vi "storeADCMixedToArray-vphil.vi"(2 "dataBlockArray1":string[](array[string]), 3 "ADCselect":enum16{"ADC18", "ADC16", "2ADC", "None"}(ring)) -> (0 "ADC16Resets":i32, 1 "TotalTrigger":i32)   [LabVIEW 2014]
uses:
  Global 1.vi
panel:
  out "ADC18Resets":i32
  out "ADC18Counter":i32
  out "ADC16Counter":i32
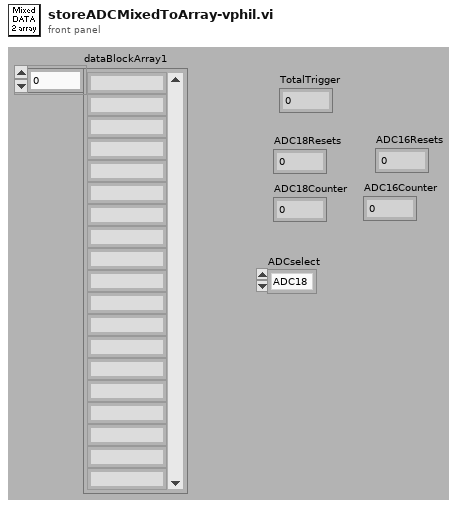
[diagram p1: front panel]
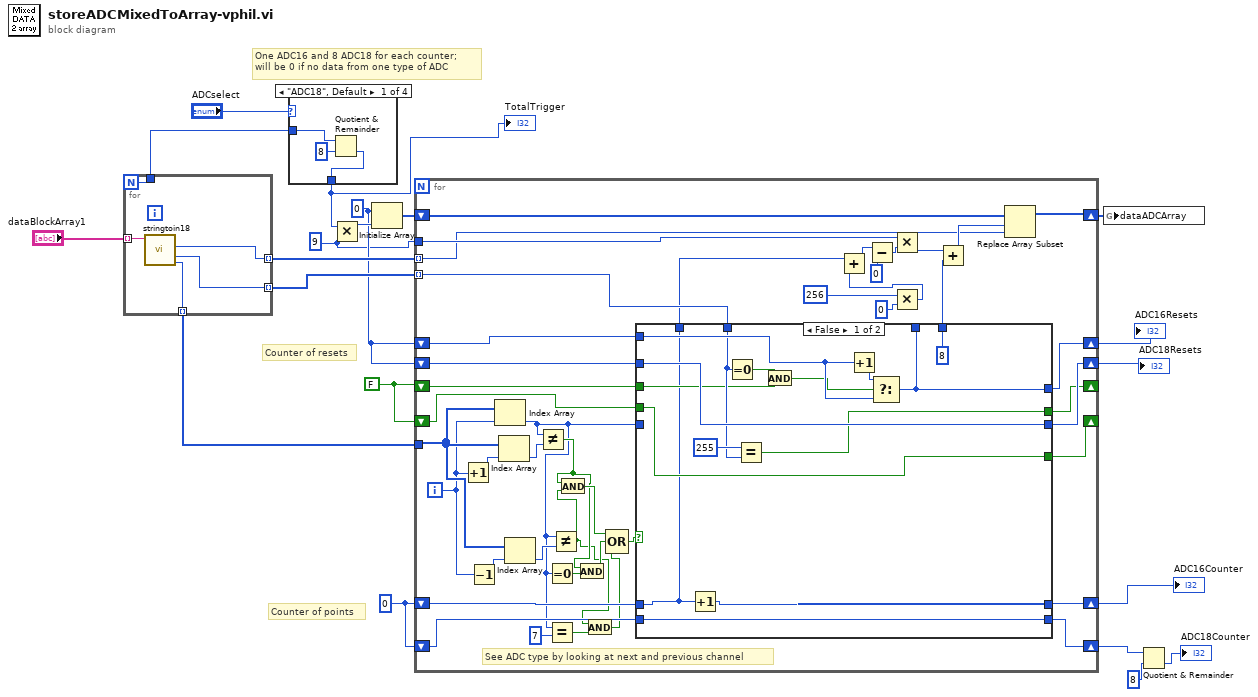
[diagram p0: block diagram]
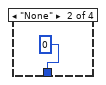
[diagram p2: hidden frame]
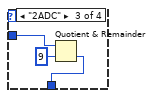
[diagram p3: hidden frame]
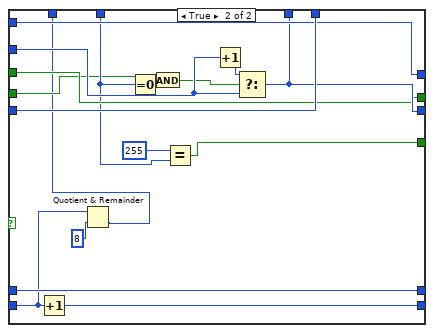
[diagram p5: hidden frame]
diagram:
  w2 = FALSE
  w9 = 0
  w1 = 9 ("dimension size")
  w4 = 0
  # "Counter of points"
  # "Counter of resets"
  # "One ADC16 and 8 ADC18 for each counter;\nwill be 0 if no data from one type of ADC"
  n1 = for {
    N -> [w21]
    tunnel: "dataBlockArray1" -> [w25] mode=indexing
    tunnel: [w24] -> w11 mode=indexing
    tunnel: [w23] -> w12 mode=indexing
    tunnel: [w22] -> w18 mode=indexing
    tunnel: [w21] -> w14
    n2 = call "stringtoin18.vi"("input_string"=w25) -> ("channel"=w22:u8, "counter"=w24:u8, "outputComplemented_int"=w23:i32)  [unwired: 8 out]
  }
  n3 = case shown="\"ADC18\", Default" "ADCselect" {
    tunnel: w14 -> [w28 _ w32 w33]
    tunnel: [w26 0 w30 w33] -> w13
    frame "ADC18", Default {
      n4 = Quotient & Remainder(x=w28, y=8) -> (floor(x/y)=w26:i32)  [unwired: 1 out]
    }
    frame "None" {
    }
    frame "2ADC" {
      n5 = Quotient & Remainder(x=w32, y=9) -> (floor(x/y)=w30:i32)  [unwired: 1 out]
    }
    frame "ADC16" {
    }
  }
  "TotalTrigger" <- w13
  n6 = Multiply(x=w13, y=w1) -> (x*y=w17:i32)
  n7 = Initialize Array(w4, w17) -> (w19:i32[])
  n8 = for {
    shift-right: [w71] -> w16
    shift-left: w19 -> [w74]
    tunnel: w11 -> [w40] mode=indexing
    tunnel: w12 -> [w72] mode=indexing
    tunnel: w18 -> [w63]
    tunnel: w1 -> [w75]
    shift-right: [w43] -> w10
    shift-left: w4 -> [w46]
    shift-right: [w44] -> w3
    shift-left: w4 -> [w42]
    shift-right: [w59] -> w8
    shift-left: w9 -> [w60]
    shift-right: [w57] -> w7
    shift-left: w9 -> [w58]
    shift-right: [w38] -> _
    shift-left: w2 -> [w39]
    shift-right: [w36] -> _
    shift-left: w2 -> [w37]
    i -> [w45]
    # "See ADC type by looking at next and previous channel"
    n9 = Increment(x=w45) -> (x+1=w68:i32)
    n10 = Decrement(x=w45) -> (x-1=w65:i32)
    n11 = Index Array(array=w63, index=w45) -> (element=w41:u8)
    n12 = Index Array(array=w63, index=w68) -> (element=w76:u8)
    n13 = Index Array(array=w63, index=w65) -> (element=w64:u8)
    n14 = Not Equal?(x=w41, y=w76) -> (x != y?=w54:bool)
    n15 = Equal To 0?(x=w41) -> (x = 0?=w55:bool)
    n16 = Equal?(x=w41, y=7) -> (x = y?=w51:bool)
    n17 = Not Equal?(x=w41, y=w64) -> (x != y?=w50:bool)
    n18 = And(x=w54, y=w50) -> (x .and. y?=w62:bool)
    n19 = And(x=w54, y=w55) -> (x .and. y?=w53:bool)
    n20 = And(x=w50, y=w51) -> (x .and. y?=w49:bool)
    n21 = Compound Arithmetic op=OR(w62, w53, w49) -> (w56:bool)
    n22 = case shown="False" w56 {
      tunnel: [8 ("y") w107] -> w61
      tunnel: w60 -> [w77 w108]
      tunnel: [w78 w108] -> w59
      tunnel: w58 -> [w90 w92]
      tunnel: [w90 w94] -> w57
      tunnel: w41 -> [_ w107]
      tunnel: w46 -> [w88 w104]
      tunnel: [w87 w104] -> w43
      tunnel: [w87 w103] -> _
      tunnel: w40 -> [w82 w98]
      tunnel: [w86 w103] -> w44
      tunnel: w42 -> [w86 w105]
      tunnel: w39 -> [w81 w101]
      tunnel: [w79 w101] -> w38
      tunnel: w37 -> [w80 w96]
      tunnel: [w80 w99] -> w36
      tunnel: [w77 w93] -> w34
      frame False {
        n23 = Increment(x=w77) -> (x+1=w78:i32)
        n24 = Equal To 0?(x=w82) -> (x = 0?=w83:bool)
        n25 = Equal?(x=u8 255, y=w82) -> (x = y?=w79:bool)
        n26 = And(x=w83, y=w81) -> (x .and. y?=w84:bool)
        n27 = Increment(x=w88) -> (x+1=w89:i32)
        n28 = Select(t=w89, s=w84, f=w88) -> (s? t:f=w87:i32)
      }
      frame True {
        n29 = Increment(x=w92) -> (x+1=w94:i32)
        n30 = Quotient & Remainder(x=w92, y=8) -> (floor(x/y)=w93:i32)  [unwired: 1 out]
        n31 = Equal To 0?(x=w98) -> (x = 0?=w102:bool)
        n32 = And(x=w96, y=w102) -> (x .and. y?=w97:bool)
        n33 = Equal?(x=u8 255, y=w98) -> (x = y?=w99:bool)
        n34 = Increment(x=w105) -> (x+1=w106:i32)
        n35 = Select(t=w106, s=w97, f=w105) -> (s? t:f=w103:i32)
      }
    }
    n36 = Multiply(x=256, y=0) -> (x*y=w47:i32)
    n37 = Add(x=w34, y=w47) -> (x+y=w70:i32)
    n38 = Subtract(x=w70, y=0) -> (x-y=w67:i32)
    n39 = Multiply(x=w75, y=w67) -> (x*y=w69:i32)
    n40 = Add(x=w69, y=w61) -> (x+y=w73:i32)
    n41 = Replace Array Subset(array=w74, new element=w72, index=w73) -> (w71:i32[])
  }
  "ADC16Resets" <- w10
  "ADC16Counter" <- w8
  "ADC18Resets" <- w3
  n42 = global write "Global 1.vi" "dataADCArray"(w16) -> ()
  n43 = Quotient & Remainder(x=w7, y=8) -> (floor(x/y)=→"ADC18Counter":i32)  [unwired: 1 out]
